vi "RFSG Pulsed Data.vi"() -> ()   [LabVIEW 2023]
doc: "Demonstrates how to use scripts to generate pulsed data. Pulsed data is typically used in time division multiplexing (TDM) systems. TDM is a type of multiplexing where two or more channels of information are transmitted over the same link by allocating a different time interval (\"slot\") for the transmission of each channel. The set of all slots makes up a frame. This example generates a CW inside one of the time slots."
uses:
  <vilib>/Utility/error.llb/DialogType.ctl
  <instrlib>/niRFSG/niRFSG.llb/niRFSG Signal Names.ctl
  <instrlib>/niRFSG/niRFSG.llb/niRFSG Signal Identifiers.ctl
  <instrlib>/niRFSG/niRFSG.llb/niRFSG Exported Signal Destinations.ctl
  <instrlib>/niRFSG/niRFSG.llb/niRFSG Write Arb Waveform (I-Q).vi
panel:
  out "Error Out":errorcluster
  in  "Resource Name":refnum<k15>="5842_0" caption="resource name"
  in  "Frame Period (s)":dbl=0.0001 format="%_3p"
  out "Actual Time Slot Period (s)":dbl=5e-05 format="%_3p"
  out "Actual Frame Period (s)":dbl=0.0001 format="%_3p"
  out "Actual IQ Rate (S/s)":dbl=10000000.0 format="%#.3p"
  in  "IQ Rate (S/s)":dbl=10000000.0 format="%#.3p"
  in  "Time Slots":i32=2 min=1 max=100
  in  "Stop":bool
  in  "Center Frequency (Hz)":dbl=10000000000.0 format="%#.3p"
  in  "Power Level (dBm)":dbl=-20.0 format="%_3f"
  # "Overview: Demonstrates how to use scripts to generate pulsed data. \nRequirements: NI-RFSG\nInstructions:\n1. Change the Resource Name to your device.\n2. Run the VI.\n3. Click Stop to stop the VI."
  # "In order to configure new settings you must stop the example using \nthe Stop button and then run the example with the new settings."
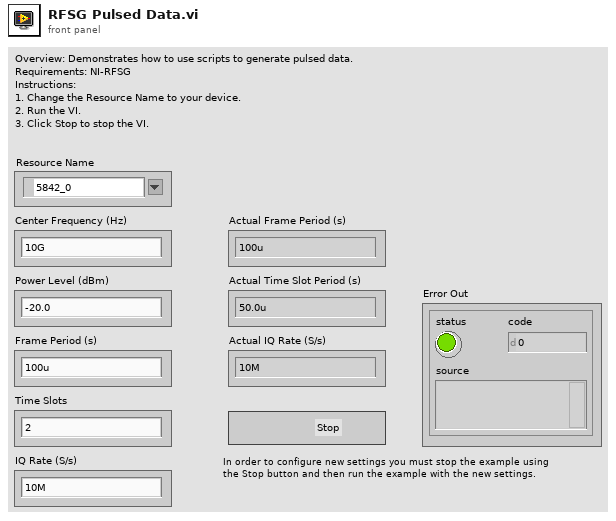
[diagram p1: front panel]
types:
  T1 = typedef "niRFSG Exported Signal Destinations.ctl" = string
  T2 = typedef "niRFSG Signal Identifiers.ctl" = string
  T3 = typedef "niRFSG Signal Names.ctl" = i32
  T4 = typedef "DialogType.ctl" = u16
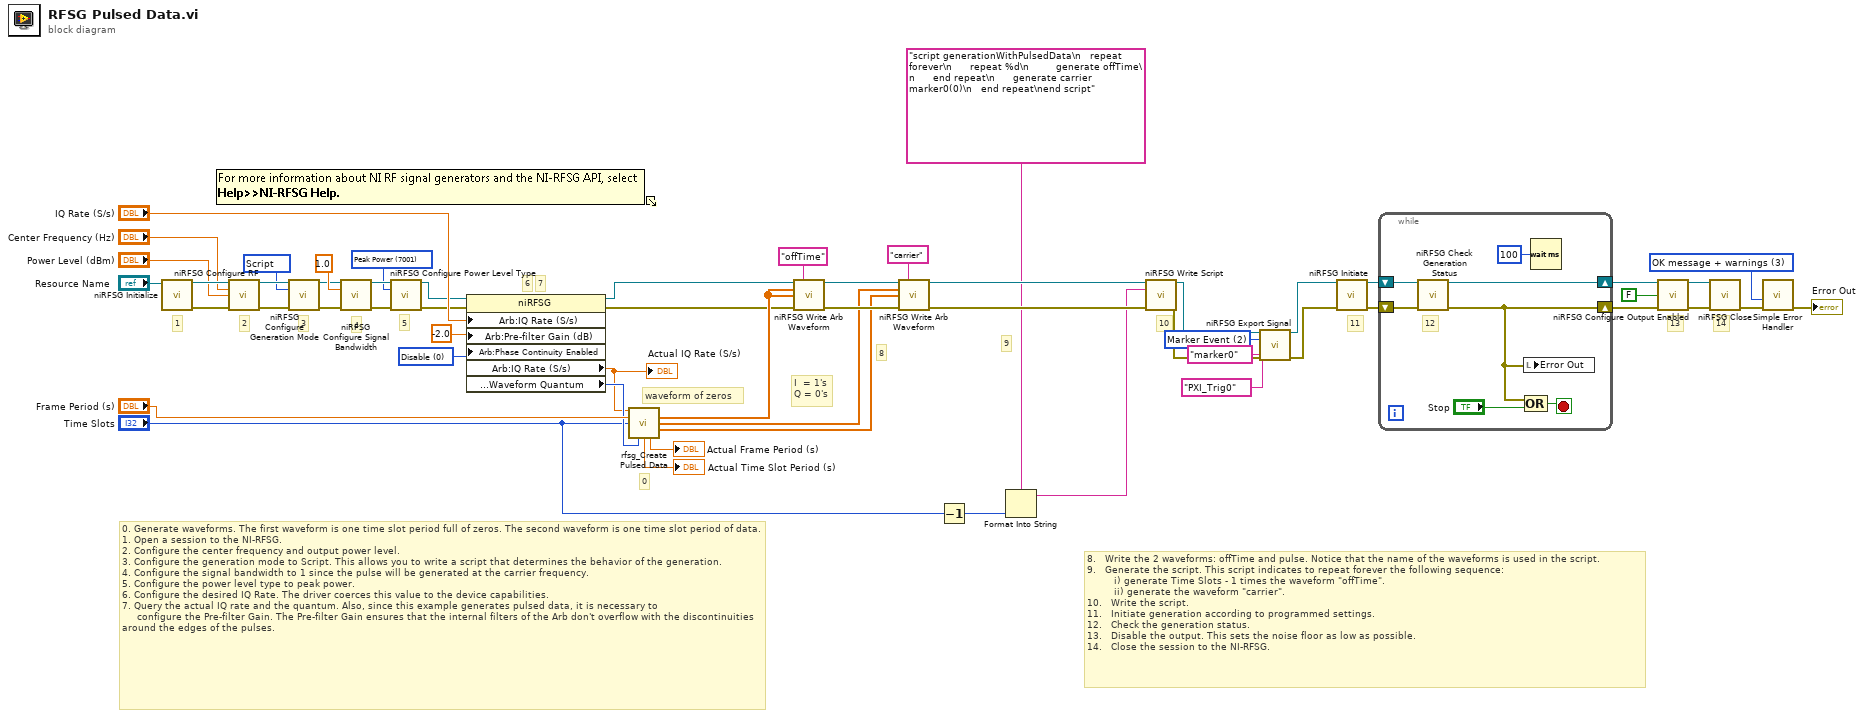
[diagram p0: block diagram]
diagram:
  w3 = T3 2 items=["Start Trigger", "Script Trigger", "Marker Event", "Ref Clock", "Started Event", "Done Event", "Configuration List Step Trigger", "Configuration Settled Event"] ("signal")
  w14 = T4 3 items=["no dialog", "OK message", "continue or stop message", "OK message + warnings", "continue/stop + warnings"] ("type of dialog (OK msg:1)")
  w15 = 7001 items=["Average Power"=7000, "Peak Power"=7001] ("power level type")
  w28 = 0 items=["Auto"=-1, "Disable"=0, "Enable"=1] ("Arb Waveform:Phase Continuity Enabled")
  w39 = 1002 items=["CW"=1000, "Arb Waveform"=1001, "Script"=1002] ("generation mode")
  # "I  = 1's\nQ = 0's"
  # "8"
  # "waveform of zeros"
  # "5"
  # "4"
  # "9"
  # "7"
  # "6"
  # "8.   Write the 2 waveforms: offTime and pulse. Notice that the name of the waveforms is used in the script.\n9.   Generate the script. This script indicates to repeat forever the following sequence:\n         i) generate Time Slots - 1 times the waveform \"offTime\".\n         ii) generate the waveform \"carrier\". \n10.   Write the script. \n11.   Initiate generation according to programmed settings.\n12.   Check the generation status.\n13.   Disable the output. This sets the noise floor as low as possible.\n14.   Close the session to the NI-RFSG."
  # "0"
  # "0. Generate waveforms. The first waveform is one time slot period full of zeros. The second waveform is one time slot period of data.\n1. Open a session to the NI-RFSG.\n2. Configure the center frequency and output power level.\n3. Configure the generation mode to Script. This allows you to write a script that determines the behavior of the generation.\n4. Configure the signal bandwidth to 1 since the pulse will be generated at the carrier frequency.\n5. Configure the power level type to peak power.\n6. Configure the desired IQ Rate. The driver coerces this value to the device capabilities.\n7. Query the actual IQ rate and the quantum. Also, since this example generates pulsed data, it is necessary to \n     configure the Pre-filter Gain. The Pre-filter Gain ensures that the internal filters of the Arb don't overflow with the discontinuities around the edges of the pulses."
  # "14"
  # "11"
  # "10"
  # "3"
  # "2"
  # "1"
  # "13"
  n1 = call <instrlib>:"niRFSG Initialize.vi"("resource name"="Resource Name") -> ("instrument handle"=w56:refnum<k15>, "error out"=w55:errorcluster)  [unwired: 13 in]
  n2 = call <instrlib>:"niRFSG Configure RF.vi"("instrument handle"=w56, "frequency (Hz)"="Center Frequency (Hz)", "power level (dBm)"="Power Level (dBm)", "error in"=w55) -> ("instrument handle out"=w54:refnum<k15>, "error out"=w53:errorcluster)  [unwired: 10 in]
  n3 = call <instrlib>:"niRFSG Configure Generation Mode.vi"("instrument handle"=w54, "generation mode"=w39, "error in"=w53) -> ("instrument handle out"=w23:refnum<k15>, "error out"=w22:errorcluster)  [unwired: 11 in]
  n4 = call <instrlib>:"niRFSG Configure Signal Bandwidth.vi"("instrument handle"=w23, "signal bandwidth (Hz)"=1.0 ("x"), "error in"=w22) -> ("instrument handle out"=w19:refnum<k15>, "error out"=w17:errorcluster)  [unwired: 11 in]
  n5 = call <instrlib>:"niRFSG Configure Power Level Type.vi"("instrument handle"=w19, "power level type"=w15, "error in"=w17) -> ("instrument handle out"=w18:refnum<k15>, "error out"=w16:errorcluster)  [unwired: 11 in]
  n6 = property class="niRFSG"(reference=w18, error in=w16, "Arb:IQ Rate (S/s)"="IQ Rate (S/s)", "Arb:Pre-filter Gain (dB)"=-2.0 ("RF:Advanced:AWG:DUC Pre-filter Gain (dB)"), "Arb:Phase Continuity Enabled"=w28) -> (reference out=w20:refnum<k15>, error out=w21:errorcluster, "Arb:IQ Rate (S/s)"=w29:dbl, "Arb:Waveform Capabilities:Waveform Quantum"=w30:i32)
  "Actual IQ Rate (S/s)" <- w29
  n7 = call <instrlib>:"rfsg_Create Pulsed Data.vi"("Sample Rate (S/s)"=w29, "Frame Period (s)"="Frame Period (s)", "Time Slots"="Time Slots", "Quantum"=w30) -> ("off Data"=w38:dbl[], "I Data"=w37:dbl[], "Q Data"=w36:dbl[], "Actual Time Slot Period (s)"=→"Actual Time Slot Period (s)":dbl, "Actual Frame Period (s)"=→"Actual Frame Period (s)":dbl)  [unwired: 7 in]
  n8 = call-poly <instrlib>:"niRFSG Write Arb Waveform.vi"("instrument handle"=w20, "name"="offTime", "I Data"=w38, "Q Data"=w38, "error in"=w21) -> ("instrument handle out"=w43:refnum<k15>, "error out"=w42:errorcluster)  [unwired: 9 in]
  n9 = call-poly <instrlib>:"niRFSG Write Arb Waveform.vi"("instrument handle"=w43, "name"="carrier", "I Data"=w37, "Q Data"=w36, "error in"=w42) -> ("instrument handle out"=w41:refnum<k15>, "error out"=w40:errorcluster)  [unwired: 9 in]
  n10 = Decrement(x="Time Slots") -> (x-1=w8:i32)
  n11 = Format Into String(format string="script generationWithPulsedData\n   repeat forever\n      repeat %d\n         generate offTime\n      end repeat\n      generate carrier marker0(0)\n   end repeat\nend script" ("script"), w8) -> (resulting string=w31:string)  [unwired: 2 in, 1 out]
  n12 = call <instrlib>:"niRFSG Write Script.vi"("instrument handle"=w41, "script"=w31, "error in"=w40) -> ("instrument handle out"=w7:refnum<k15>, "error out"=w6:errorcluster)  [unwired: 11 in]
  n13 = call <instrlib>:"niRFSG Export Signal.vi"("instrument handle"=w7, "signal"=w3, "signal identifier"=T2 "marker0", "output terminal"=T1 "PXI_Trig0", "error in"=w6) -> ("instrument handle out"=w5:refnum<k15>, "error out"=w4:errorcluster)  [unwired: 9 in]
  n14 = call <instrlib>:"niRFSG Initiate.vi"("instrument handle"=w5, "error in"=w4) -> ("instrument handle out"=w52:refnum<k15>, "error out"=w11:errorcluster)  [unwired: 12 in]
  n15 = while {
    shift-right: [w62] -> w46
    shift-left: w52 -> [w63]
    shift-right: [w57] -> w12
    shift-left: w11 -> [w58]
    stop <- w61 stop-if-true
    # "12"
    n16 = call <instrlib>:"niRFSG Check Generation Status.vi"("instrument handle"=w63, "error in"=w58) -> ("instrument handle out"=w62:refnum<k15>, "error out"=w57:errorcluster)  [unwired: 11 in, 1 out]
    n17 = local write "Error Out"(w57) -> ()
    n18 = Compound Arithmetic op=OR(w57, "Stop") -> (w61:bool)
    n19 = Wait (ms)(milliseconds to wait=u32 100) -> ()  [unwired: 1 out]
  }
  n20 = call <instrlib>:"niRFSG Configure Output Enabled.vi"("instrument handle"=w46, "output enabled"=FALSE ("output enable"), "error in"=w12) -> ("instrument handle out"=w47:refnum<k15>, "error out"=w45:errorcluster)  [unwired: 11 in]
  n21 = call <instrlib>:"niRFSG Close.vi"("instrument handle"=w47, "error in"=w45) -> ("error out"=w13:errorcluster)  [unwired: 13 in]
  n22 = call <vilib>:"Simple Error Handler.vi"("type of dialog (OK msg:1)"=w14, "error in (no error)"=w13) -> ("error out"=→"Error Out":errorcluster)  [unwired: 3 in, 4 out]
